vi "Mean PtByPt.vi"(0 "x":dbl format="%0.2f", 1 "sample length":i32=100, 2 "initialize":bool) -> (3 "mean":dbl format="%0.2f", 5 "error":i32)   [LabVIEW 2017, in "NI_PtbyPt.lvlib"]
doc: "Computes the <B>mean</B>, or average, of the values in the set of input data points specified by <B>sample length</B>. If the number of values is less than the <B>sample length</B>, the VI uses the number of values to compute the mean."
uses:
  <vilib>/ptbypt/NI_PtbyPt.lvlib
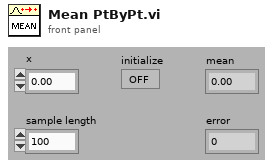
[diagram p1: front panel]
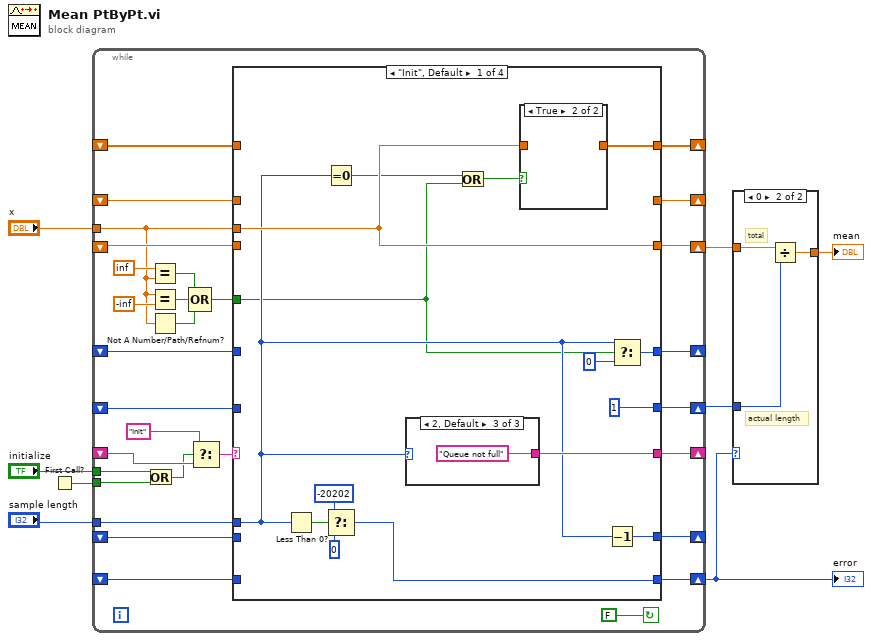
[diagram p0: block diagram]
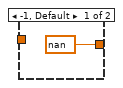
[diagram p2: hidden frame]
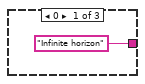
[diagram p3: hidden frame]
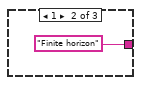
[diagram p4: hidden frame]
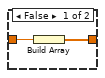
[diagram p5: hidden frame]
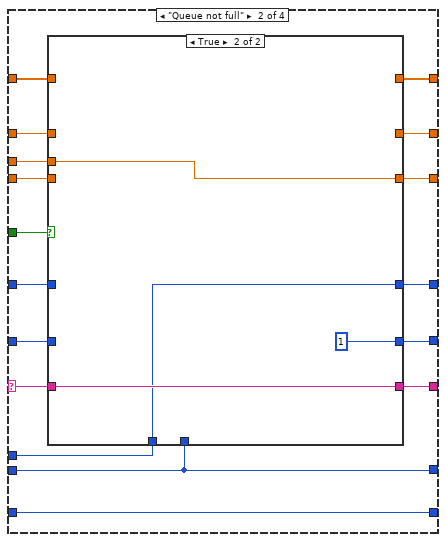
[diagram p6: hidden frame]
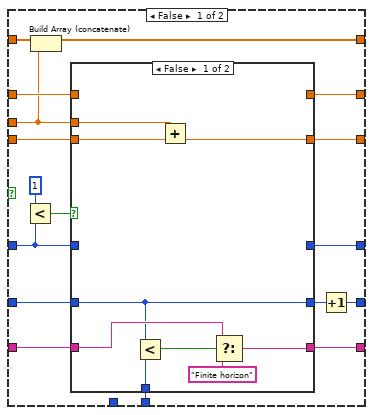
[diagram p7: hidden frame]
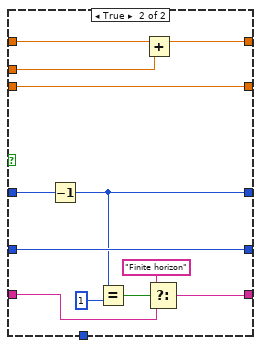
[diagram p8: hidden frame]
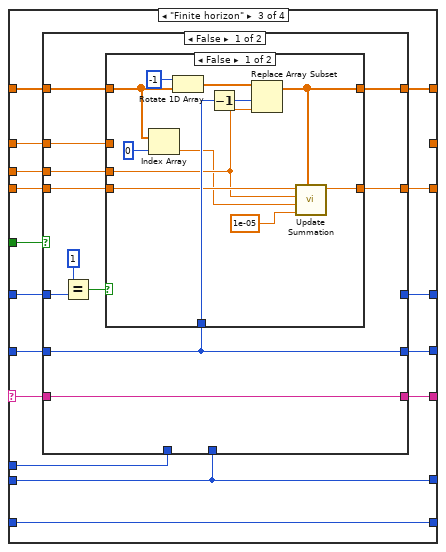
[diagram p9: hidden frame]
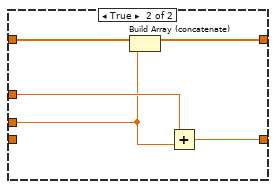
[diagram p10: hidden frame]
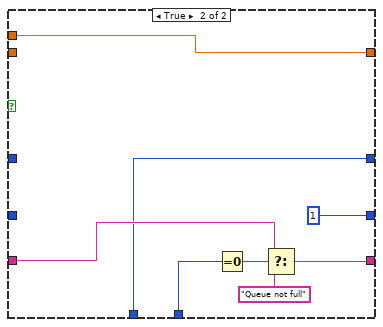
[diagram p11: hidden frame]
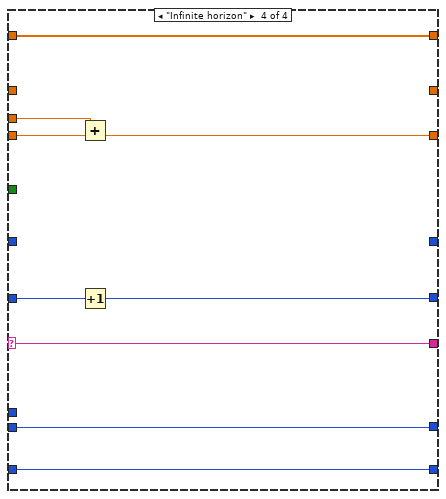
[diagram p12: hidden frame]
diagram:
  n1 = First Call?() -> (First Call?: T/F=w5:bool)
  n2 = while {
    tunnel: w5 -> [w10]
    shift-left: _ -> [w27]
    shift-right: [w28] -> _
    shift-left: _ -> [w30]
    shift-right: [w29] -> _
    shift-left: _ -> [w32]
    shift-right: [w33] -> w6
    shift-left: _ -> [w34]
    shift-right: [w35] -> w7
    shift-left: _ -> [w38]
    shift-right: [w31] -> _
    shift-right: [w18] -> _
    shift-left: _ -> [w17]
    shift-right: [w16] -> _
    shift-left: _ -> [w15]
    shift-right: [w14] -> w4
    shift-left: _ -> [w13]
    tunnel: "x" -> [w12]
    tunnel: "sample length" -> [w11]
    tunnel: "initialize" -> [w9]
    stop <- FALSE continue-if-true
    n3 = Or(x=w9, y=w10) -> (x .or. y?=w25:bool)
    n4 = Equal?(x=inf, y=w12) -> (x = y?=w21:bool)
    n5 = Equal?(x=w12, y=-inf) -> (x = y?=w22:bool)
    n6 = Not A Number/Path/Refnum?(number/path/refnum=w12) -> (NaN/Path/Refnum?=w20:bool)
    n7 = Compound Arithmetic op=OR(w21, w22, w20) -> (w19:bool)
    n8 = Select(t="Init", s=w25, f=w38) -> (s? t:f=w36:string)
    n9 = case shown="\"Init\", Default" w36 {
      selector: w36 -> [_ w68 w123 w174]
      tunnel: [w44 w71 w130 w176] -> w35
      tunnel: w34 -> [_ w72 w129 w178]
      tunnel: w12 -> [w44 w73 w133 w177]
      tunnel: [1 w70 w120 w170] -> w33
      tunnel: w32 -> [_ w69 w124 w175]
      tunnel: [w42 w67 w122 w174] -> w31
      tunnel: w30 -> [_ w75 w131 w173]
      tunnel: [w43 w74 w132 w173] -> w29
      tunnel: w11 -> [w41 w60 w119 _]
      tunnel: [w48 w66 w121 w172] -> w28
      tunnel: w27 -> [_ w66 w121 w172]
      tunnel: w19 -> [w40 w64 w126 _]
      tunnel: [w50 w65 w125 _] -> w18
      tunnel: w17 -> [_ w63 w128 _]
      tunnel: [_ w62 _ _] -> w16
      tunnel: w15 -> [_ w61 w127 _]
      tunnel: [w46 w59 w118 w171] -> w14
      tunnel: w13 -> [_ w59 w118 w171]
      frame "Init", Default {
        n10 = Less Than 0?(x=w41) -> (x < 0?=w51:bool)
        n11 = Equal To 0?(x=w41) -> (x = 0?=w39:bool)
        n12 = Select(t=-20202, s=w51, f=0) -> (s? t:f=w46:i32)
        n13 = case shown="2, Default" w41 {
          tunnel: ["Infinite horizon" "Finite horizon" "Queue not full" ("f")] -> w42
          frame 0 {
          }
          frame 1 {
          }
          frame 2, Default {
          }
        }
        n14 = Or(x=w39, y=w40) -> (x .or. y?=w45:bool)
        n15 = case shown="True" w45 {
          tunnel: w44 -> [w58 _]
          tunnel: [w57 _] -> w43
          frame False {
            n16 = Build Array(w58) -> (w57:dbl[])
          }
          frame True {
          }
        }
        n17 = Decrement(x=w41) -> (x-1=w48:i32)
        n18 = Select(t=w41, s=w40, f=0) -> (s? t:f=w50:i32)
      }
      frame "Queue not full" {
        n19 = case shown="True" w64 {
          tunnel: w75 -> [w85 _]
          tunnel: [w83 _] -> w74
          tunnel: w73 -> [w82 w117]
          tunnel: w72 -> [w92 _]
          tunnel: [w91 w117] -> w71
          tunnel: [w79 1] -> w70
          tunnel: w69 -> [w90 _]
          tunnel: w68 -> [w89 w115]
          tunnel: [w88 w115] -> w67
          tunnel: w66 -> [w87 _]
          tunnel: [w81 w114] -> w65
          tunnel: w63 -> [w78 _]
          tunnel: [w86 _] -> w62
          tunnel: w61 -> [w84 _]
          tunnel: w60 -> [_ w114]
          frame False {
            n20 = Less?(x=1, y=w78) -> (x < y?=w76:bool)
            n21 = Build Array (concatenate)(w85, w82) -> (w83:dbl[])
            n22 = case shown="False" w76 {
              tunnel: w82 -> [w101 w113]
              tunnel: w92 -> [w100 w106]
              tunnel: [w99 w106] -> w91
              tunnel: [w93 w104] -> w80
              tunnel: w90 -> [w93 w104]
              tunnel: w89 -> [w98 w108]
              tunnel: [w97 w109] -> w88
              tunnel: w87 -> [w96 _]
              tunnel: w84 -> [_ w105]
              tunnel: [_ w112] -> w86
              tunnel: w78 -> [_ w111]
              tunnel: [_ w103] -> w81
              frame False {
                n23 = Less?(x=w93, y=w96) -> (x < y?=w95:bool)
                n24 = Add(x=w101, y=w100) -> (x+y=w99:dbl)
                n25 = Select(t=w98, s=w95, f="Finite horizon") -> (s? t:f=w97:string)
              }
              frame True {
                n26 = Decrement(x=w111) -> (x-1=w103:i32)
                n27 = Equal?(x=w103, y=1) -> (x = y?=w110:bool)
                n28 = Add(x=w105, y=w113) -> (x+y=w112:dbl)
                n29 = Select(t="Finite horizon" ("f"), s=w110, f=w108) -> (s? t:f=w109:string)
              }
            }
            n30 = Increment(x=w80) -> (x+1=w79:i32)
          }
          frame True {
          }
        }
      }
      frame "Finite horizon" {
        n31 = case shown="False" w126 {
          tunnel: w133 -> [w144 w169]
          tunnel: [w143 _] -> w132
          tunnel: w131 -> [w142 _]
          tunnel: [w141 w169] -> w130
          tunnel: w129 -> [w137 _]
          tunnel: w128 -> [w136 _]
          tunnel: w127 -> [w140 _]
          tunnel: [_ w162] -> w125
          tunnel: w124 -> [w138 _]
          tunnel: w123 -> [w139 w164]
          tunnel: [w139 w165] -> w122
          tunnel: w121 -> [_ w163]
          tunnel: [w138 1] -> w120
          tunnel: w119 -> [_ w162]
          frame False {
            n32 = Equal?(x=1, y=w136) -> (x = y?=w134:bool)
            n33 = case shown="False" w134 {
              tunnel: w144 -> [w147 w157]
              tunnel: w138 -> [w152 _]
              tunnel: [w148 w160] -> w143
              tunnel: w142 -> [w151 w159]
              tunnel: [w149 w161] -> w141
              tunnel: w137 -> [w150 _]
              tunnel: w140 -> [_ w158]
              frame False {
                n34 = Index Array(array=w151, index=0 ("Index")) -> (element=w146:dbl)
                n35 = Rotate 1D Array(1:w151, 2:i16 -1 ("n")) -> (0:w154:dbl[])
                n36 = Decrement(x=w152) -> (x-1=w153:i32)
                n37 = Replace Array Subset(array=w154, new element=w147, index=w153) -> (w148:dbl[])
                n38 = call <vilib>:"Update Summation.vi"("Data Set"=w148, "tolerance"=1e-05, "x0"=w146, "x"=w147, "summation in"=w150) -> ("summation out"=w149:dbl)  [unwired: 6 out]
              }
              frame True {
                n39 = Build Array (concatenate)(w159, w157) -> (w160:dbl[])
                n40 = Add(x=w158, y=w157) -> (x+y=w161:dbl)
              }
            }
          }
          frame True {
            n41 = Equal To 0?(x=w163) -> (x = 0?=w167:bool)
            n42 = Select(t=w164, s=w167, f="Queue not full") -> (s? t:f=w165:string)
          }
        }
      }
      frame "Infinite horizon" {
        n43 = Add(x=w177, y=w178) -> (x+y=w176:dbl)
        n44 = Increment(x=w175) -> (x+1=w170:i32)
      }
    }
  }
  "error" <- w4
  n45 = case shown="0" w4 {
    tunnel: [nan w182] -> w8
    tunnel: w7 -> [_ w181]
    tunnel: w6 -> [_ w180]
    frame -1, Default {
    }
    frame 0 {
      # "actual length"
      # "total"
      n46 = Divide(x=w181, y=w180) -> (x/y=w182:dbl)
    }
  }
  "mean" <- w8
